vi "Delete Deprecated Channels.vi"(8 "error in (no error)":errorcluster, 10 "VCOM Signal Map In":map{string, T1}(c390), 11 "System Definition File Path":path=path "C:/Users/Nick/Desktop/VCOM Config System Definition Utility/VeriStand Example Project/Example Project/Example Project.nivssdf") -> (0 "error out":errorcluster, 3 "Log":string[](array[string]))   [LabVIEW 2025]
uses:
  <vilib>/Vehicle Communication Toolkit/TypDefs/RBS Signal.ctl
  NationalInstruments.VeriStand.SystemDefinitionAPI
  <vilib>/NI/NI VeriStand Advanced SysDef API/_SubVIs/SysDef.Search.GUIDs.vi
  NationalInstruments.VeriStand.SystemStorage
  <vilib>/NI/NI VeriStand Advanced SysDef API/SysDef API/Advanced System Definition.lvlib
  <vilib>/Vehicle Communication Toolkit/Vehicle Communication Toolkit.lvlib
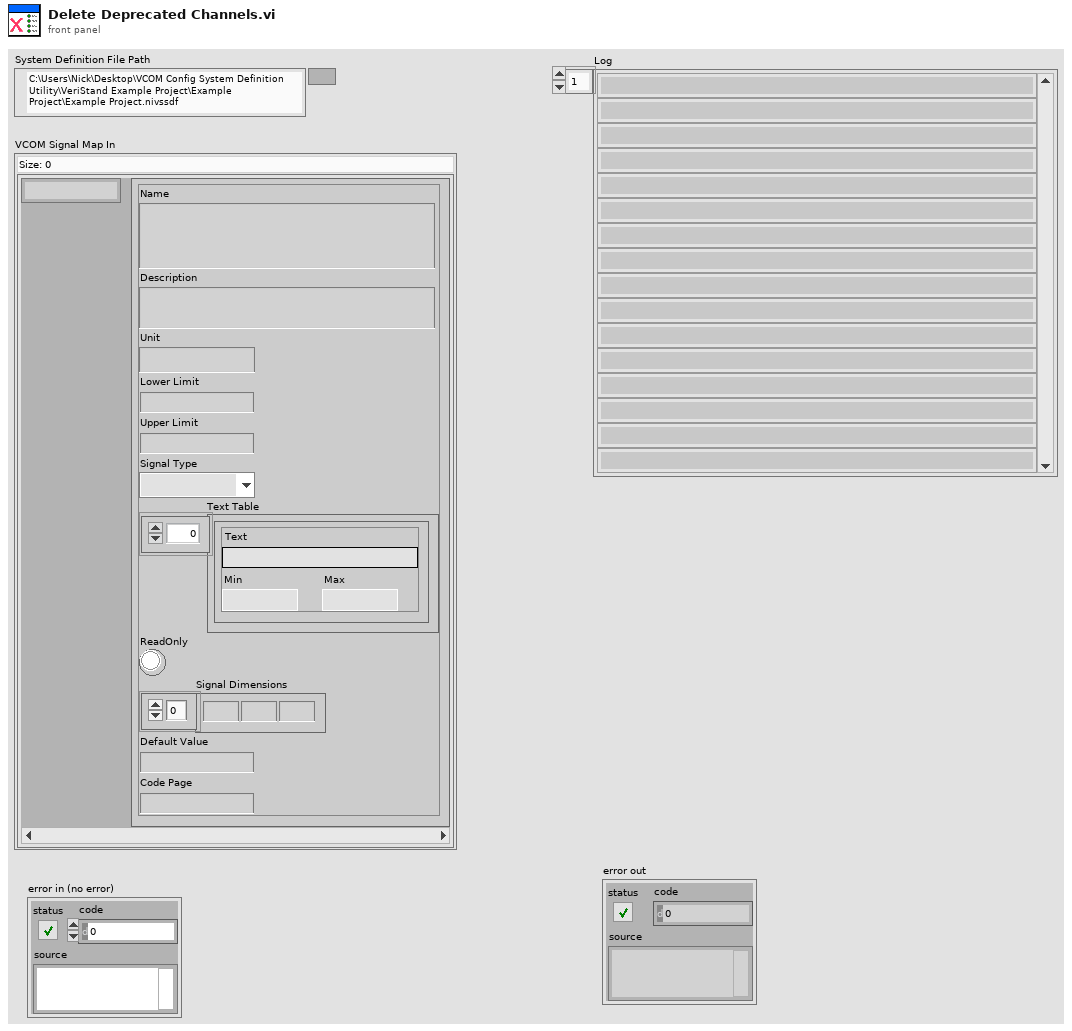
[diagram p1: front panel]
types:
  T1 = typedef "Vehicle Communication Toolkit.lvlib/RBS Signal.ctl" = cluster{"Name":string, "Description":string, "Unit":string, "Lower Limit":dbl, "Upper Limit":dbl, "Signal Type":enum32{"RE_BOOL", "RE_UINT8", "RE_INT8", "RE_UINT16", "RE_INT16", "RE_UINT32", "RE_INT32", "RE_UINT64", "RE_INT64", "RE_FLOAT32", "RE_FLOAT64", "RE_TEXT"}, "Text Table":cluster{"Text":string, "Min":dbl, "Max":dbl}[], "ReadOnly":bool, "Signal Dimensions":u32[], "Default Value":dbl, "Code Page":u32}
  T2 = typedef "Custom Device API.lvlib/Custom Device Pointer.ctl" = refnum<k24>
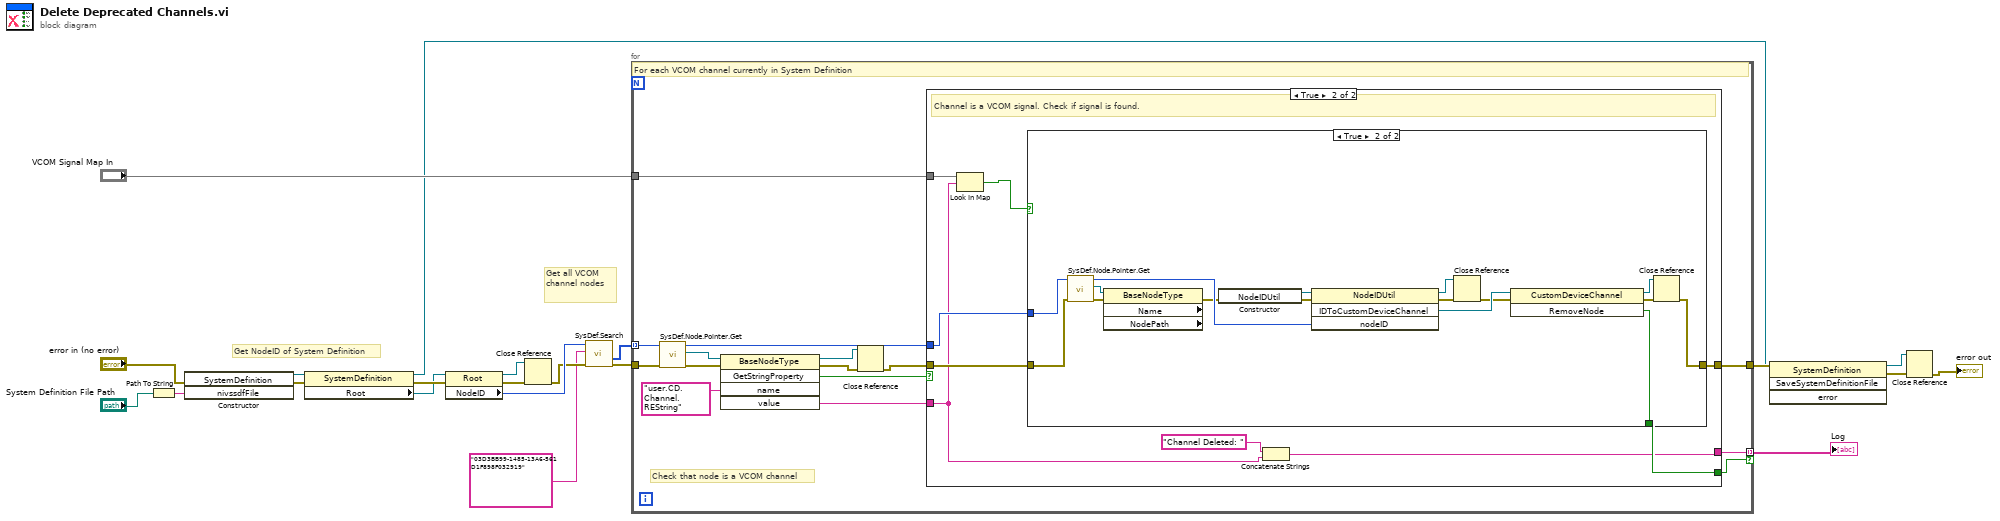
[diagram p0: block diagram]
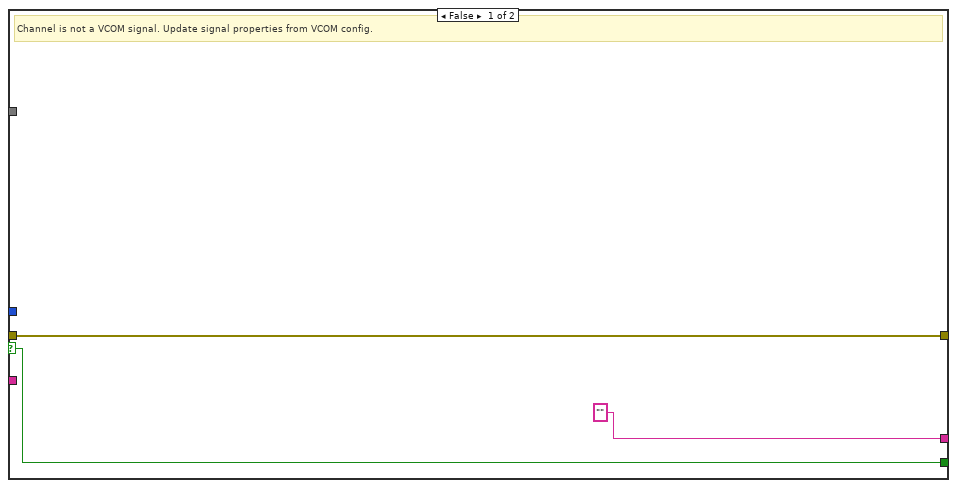
[diagram p2: hidden frame]
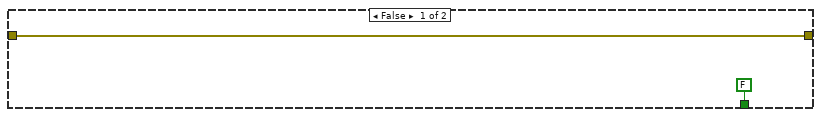
[diagram p3: hidden frame]
diagram:
  # "Get all VCOM channel nodes"
  # "Get NodeID of System Definition"
  n1 = Path To String(path="System Definition File Path") -> (string=w19:string)
  n2 = constructor class="SystemDefinition"(error in="error in (no error)", "nivssdfFile"=w19) -> (reference out=w17:refnum<k24>, error out=w18:errorcluster)  [unwired: 2 in, 2 out]
  n3 = property class="SystemDefinition"(reference=w17, error in=w18) -> (reference out=w4:refnum<k24>, error out=w15:errorcluster, "Root"=w7:refnum<k24>)
  n4 = property class="Root"(reference=w7, error in=w15) -> (reference out=w12:refnum<k24>, error out=w13:errorcluster, "NodeID"=w14:u64)
  n5 = Close Reference(reference=w12, error in (no error)=w13) -> (error out=w11:errorcluster)
  n6 = call-poly <vilib>:"SysDef.Search.vi"("error in (no error)"=w11, "GUID"="03D3BB99-1485-13A6-561D1F898F032919", "nodeID"=w14) -> ("error out"=w21:errorcluster, "Values Out"=w20:u64[])  [unwired: 5 in, 2 out]
  n7 = for {
    tunnel: w20 -> [w30] mode=indexing
    tunnel: "VCOM Signal Map In" -> [w32]
    tunnel: w21 -> [w34]
    tunnel: [w28] -> w5
    tunnel: [w26] -> w6 mode=indexing if=w22
    # "Check that node is a VCOM channel"
    # "For each VCOM channel currently in System Definition"
    n8 = call <vilib>:"SysDef.Node.Pointer.Get.vi"("error in (no error)"=w34, "nodeID"=w30) -> ("error out"=w33:errorcluster, "Node Pointer"=w36:T2, "nodeID out"=w29:u64)  [unwired: 6 in, 1 out]
    n9 = invoke class="BaseNodeType" method="GetStringProperty"(reference=w36, error in=w33, "name"="user.CD.Channel.REString") -> (reference out=w24:T2, error out=w25:errorcluster, "GetStringProperty"=w27:bool, "value"=w31:string)  [unwired: 2 in, 1 out]
    n10 = Close Reference(reference=w24, error in (no error)=w25) -> (error out=w23:errorcluster)
    n11 = case shown="True" w27 {
      selector: w27 -> [w37 _]
      tunnel: w32 -> [_ w48]
      tunnel: w31 -> [_ w40]
      tunnel: w23 -> [w39 w47]
      tunnel: w29 -> [_ w45]
      tunnel: [w39 w44] -> w28
      tunnel: ["" ("value") w41] -> w26
      tunnel: [w37 w43] -> w22
      frame False {
        # "Channel is not a VCOM signal. Update signal properties from VCOM config."
      }
      frame True {
        # "Channel is a VCOM signal. Check if signal is found."
        n12 = Look In Map(map=w48, key=w40) -> (key not found?=w46:bool)  [unwired: 1 in, 1 out]
        n13 = case shown="True" w46 {
          tunnel: w47 -> [w50 w66]
          tunnel: w45 -> [_ w65]
          tunnel: [w50 w64] -> w44
          tunnel: [FALSE ("RemoveNode") w51] -> w43
          frame False {
          }
          frame True {
            n14 = call <vilib>:"SysDef.Node.Pointer.Get.vi"("error in (no error)"=w66, "nodeID"=w65) -> ("error out"=w60:errorcluster, "Node Pointer"=w61:T2, "nodeID out"=w59:u64)  [unwired: 6 in, 1 out]
            n15 = property class="BaseNodeType" props=["Name", "NodePath"](reference=w61, error in=w60) -> (error out=w56:errorcluster)  [unwired: 3 out]
            n16 = constructor class="NodeIDUtil"(error in=w56) -> (reference out=w55:refnum<k24>, error out=w57:errorcluster)  [unwired: 2 in, 1 out]
            n17 = invoke class="NodeIDUtil" method="IDToCustomDeviceChannel"(reference=w55, error in=w57, "nodeID"=w59) -> (reference out=w54:refnum<k24>, error out=w53:errorcluster, "IDToCustomDeviceChannel"=w58:refnum<k24>)  [unwired: 1 in, 1 out]
            n18 = Close Reference(reference=w54, error in (no error)=w53) -> (error out=w52:errorcluster)
            n19 = invoke class="CustomDeviceChannel" method="RemoveNode"(reference=w58, error in=w52) -> (reference out=w62:refnum<k24>, error out=w63:errorcluster, "RemoveNode"=w51:bool)  [unwired: 1 in]
            n20 = Close Reference(reference=w62, error in (no error)=w63) -> (error out=w64:errorcluster)
          }
        }
        n21 = Concatenate Strings("Channel Deleted: " ("string"), w40) -> (w41:string)
      }
    }
  }
  "Log" <- w6
  n22 = invoke class="SystemDefinition" method="SaveSystemDefinitionFile"(reference=w4, error in=w5) -> (reference out=w2:refnum<k24>, error out=w3:errorcluster)  [unwired: 2 in, 2 out]
  n23 = Close Reference(reference=w2, error in (no error)=w3) -> (error out=→"error out":errorcluster)
